vi "p5.8 (hw3).vi"() -> ()   [LabVIEW 2017]
panel:
  out "Number of Guesses":dbl
  in  "Input (N)":dbl=1.0 min=1.0 max=1000.0
  # "Problem P 5.8 (HW 3)"
  # "Input N has to be greater than 0"
  # "Input N has to be less than 1000"
  # "Patrik Sokolowski"
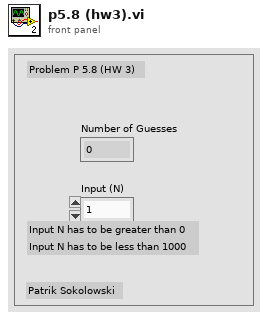
[diagram p1: front panel]
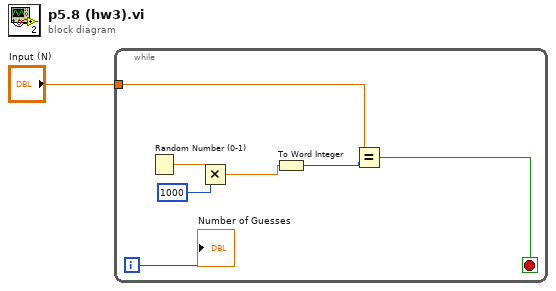
[diagram p0: block diagram]
diagram:
  n1 = while {
    tunnel: "Input (N)" -> [w7]
    i -> [w8]
    stop <- w2 stop-if-true
    n2 = Random Number (0-1)() -> (number: 0 to 1=w6:dbl)
    n3 = Multiply(x=w6, y=1000) -> (x*y=w4:dbl)
    n4 = To Word Integer(number=w4) -> (16bit integer=w3:i16)
    n5 = Equal?(x=w7, y=w3) -> (x = y?=w2:bool)
    "Number of Guesses" <- w8
  }
